vi "ReadScanFile.vi"(8 "error in":errorcluster, 10 "Header":T1, 11 "refnum in":refnum<file>) -> (0 "error out":errorcluster, 1 "Coordinate Data":dbl[][][][](array[numeric]), 2 "Scan Data":i32[][][][](array[numeric]), 3 "refnum out":refnum<file>)   [LabVIEW 2011]
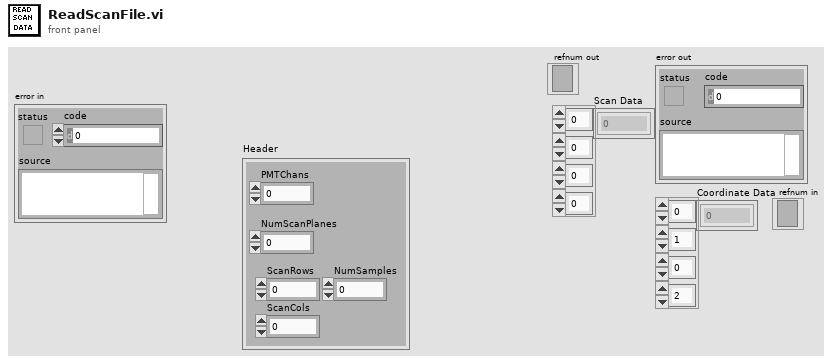
[diagram p1: front panel]
types:
  T1 = cluster{"PMTChans":i32, "NumScanPlanes":i32, "ScanRows":i32, "ScanCols":i32, "NumSamples":i32}
  T2 = enum16{"big-endian, network order", "native, host order", "little-endian"}
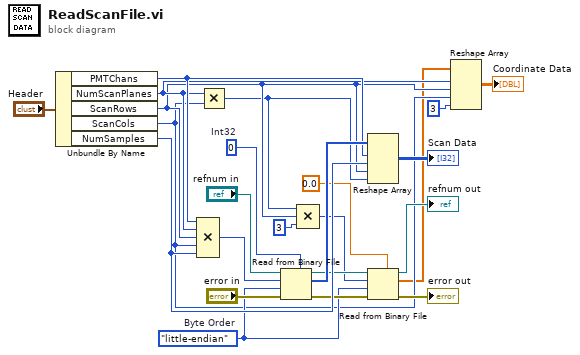
[diagram p0: block diagram]
diagram:
  w14 = T2."little-endian"  # Byte Order
  w6 = 0  # Int32
  n1 = Unbundle By Name("Header") -> ("PMTChans"=w20:i32, "NumScanPlanes"=w11:i32, "ScanRows"=w10:i32, "ScanCols"=w9:i32, "NumSamples"=w19:i32)
  n2 = Compound Arithmetic op=MULTIPLY(w20, w11, w10, w9, w19) -> (w23:i32)
  n3 = Multiply(x=w11, y=w9) -> (x*y=w1:i32)
  n4 = Read from Binary File(5:w6, 8:"error in", 9:w14, 10:w23, 11:"refnum in") -> (0:w15:errorcluster, 2:w21:i32[], 3:w17:refnum<file>)  [unwired: 1 in, 1 out]
  n5 = Compound Arithmetic op=MULTIPLY(w1, w10, 3 ("value")) -> (w16:i32)
  n6 = Reshape Array(w21, w20, w19, w10, w1) -> (→"Scan Data":i32[][][][])
  n7 = Read from Binary File(5:0.0, 8:w15, 9:w14, 10:w16, 11:w17) -> (0:→"error out":errorcluster, 2:w7:dbl[], 3:→"refnum out":refnum<file>)  [unwired: 1 in, 1 out]
  n8 = Reshape Array(w7, w11, w10, w9, 3 ("dimension size")) -> (→"Coordinate Data":dbl[][][][])
